vi "DPIDs.Initialize.vi"(8 "error in":errorcluster, 10 "UUDT Receive ID":u32=513 format="%.0x", 11 "cluster in":refnum<k21>) -> (0 "error out":errorcluster, 2 "GMLAN DPID Session":refnum<k21>, 3 "Cluster Out":refnum<k21>)   [LabVIEW 2019, in "Diagnostics Addon Engine.lvlib"]
uses:
  Diagnostics Addon Engine.lvlib
  Addon Shared/Types/XNET.Frame.ctl
  Addon Shared/Diagnostics Addon Shared.lvlib
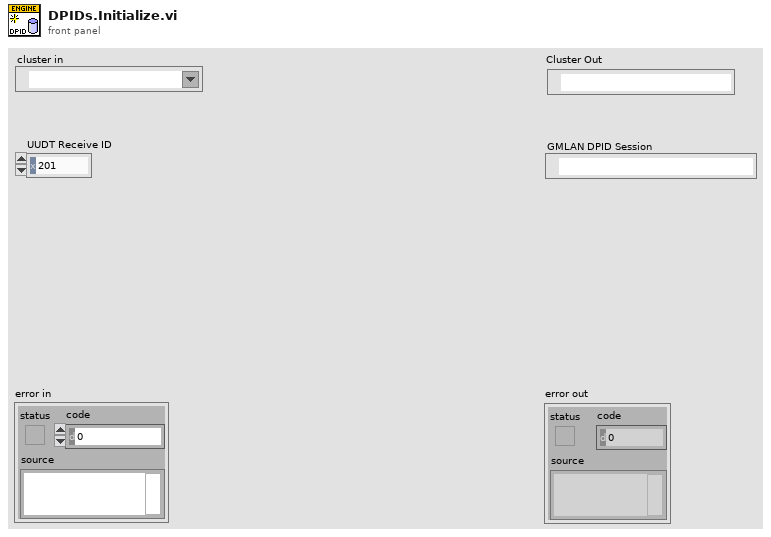
[diagram p1: front panel]
types:
  T1 = typedef "Diagnostics Addon Shared.lvlib/XNET.Frame.ctl" = cluster{"Frame name":string, "Identifier":u32, "Payload Length":u32, "Timing Type":u32, "Transmit Time":dbl, "Extended Identifier?":bool, "Comment":string}
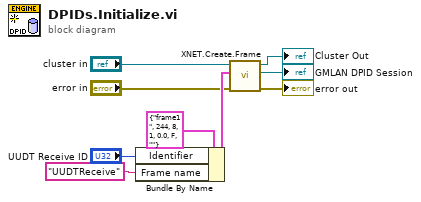
[diagram p0: block diagram]
diagram:
  n1 = Bundle By Name(cluster=T1 {"Frame name"="frame1", "Identifier"=244, "Payload Length"=8, "Timing Type"=1, "Transmit Time"=0.0, "Extended Identifier?"=FALSE, "Comment"=""} ("CAN Frame"), "Identifier"="UUDT Receive ID", "Frame name"="UUDTReceive") -> (w7:T1)
  n2 = call "XNET.Create.Frame.vi"("error in"="error in", "CAN Frame"=w7, "cluster in"="cluster in") -> ("error out"=→"error out":errorcluster, "frame out"=→"GMLAN DPID Session":refnum<k21>, "cluster out"=→"Cluster Out":refnum<k21>)  [unwired: 6 in]
